vi "Configure Power Calibration.vi"(0 "VISA resource name":refnum<visa-resource-name>, 1 "Channel (1)":i32=1, 2 "Error Correction State (F: Disabled)":bool, 3 "Port 1 (1)":i32=1, 5 "Averaging Factor (1)":i32=1, 7 "Loss Compensation (F: Disabled)":bool, 9 "Power Meter Address (1)":i32=1, 11 "error in (no error)":errorcluster) -> (4 "VISA resource name out":refnum<visa-resource-name>, 15 "error out":errorcluster)   [LabVIEW 2020, in "Agilent ENA Series.lvlib"]
doc: "Configures the power calibration settings.\n\n<b>Note:</b>\nThis VI is not supported by the E5063A model."
uses:
  <instrlib>/Agilent ENA Series/Agilent ENA Series.lvlib
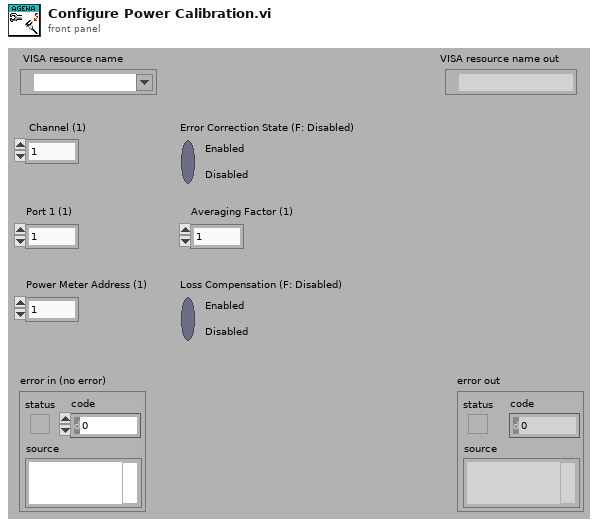
[diagram p1: front panel]
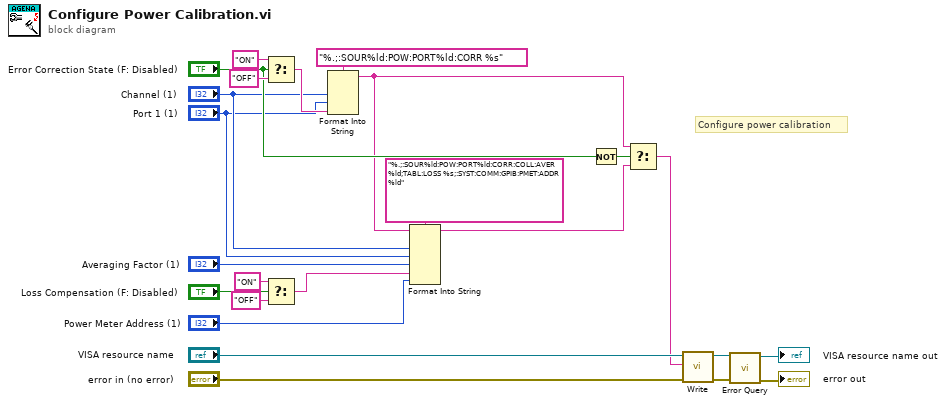
[diagram p0: block diagram]
diagram:
  # "Configure power calibration"
  n1 = Select(t="ON", s="Error Correction State (F: Disabled)", f="OFF") -> (s? t:f=w19:string)
  n2 = Select(t="ON", s="Loss Compensation (F: Disabled)", f="OFF") -> (s? t:f=w8:string)
  n3 = Format Into String(format string="%.;:SOUR%ld:POW:PORT%ld:CORR %s", "Channel (1)", "Port 1 (1)", w19) -> (resulting string=w5:string)  [unwired: 2 in, 1 out]
  n4 = Format Into String(format string="%.;:SOUR%ld:POW:PORT%ld:CORR:COLL:AVER %ld;TABL:LOSS %s;:SYST:COMM:GPIB:PMET:ADDR %ld", initial string=w5, "Channel (1)", "Port 1 (1)", "Averaging Factor (1)", w8, "Power Meter Address (1)") -> (resulting string=w15:string)  [unwired: 1 in, 1 out]
  n5 = Not(x="Error Correction State (F: Disabled)") -> (.not. x?=w17:bool)
  n6 = Select(t=w5, s=w17, f=w15) -> (s? t:f=w6:string)
  n7 = call <instrlib>:"Write.vi"("error in (no error)"="error in (no error)", "String ()"=w6, "VISA resource name"="VISA resource name") -> ("error out"=w3:errorcluster, "VISA resource name out"=w4:refnum<visa-resource-name>)  [unwired: 6 in, 1 out]
  n8 = call <instrlib>:"Error Query.vi"("error in (no error)"=w3, "VISA resource name"=w4) -> ("error out"=→"error out":errorcluster, "VISA resource name out"=→"VISA resource name out":refnum<visa-resource-name>)  [unwired: 6 in, 2 out]
